vi "GUI_Pico8752_v2.vi"() -> ()   [LabVIEW 2020]
uses:
  Shared/GUI_Template/GUI_master/tcp_new_data_event.ctl
  Shared/GUI_Template/GUI_master/tcp new data cluster.ctl
panel:
  in  "StepSize\nDogleg":dbl=10.0
  in  "StepSize\nAMP1":dbl=100.0
  in  "StepSize\nPreAmp":dbl=30.0
  in  "StepSize\nXPW":dbl=5.0
  in  "Move Device 11 Neg":bool
  in  "Move Device 11 Pos":bool
  in  "Move Device 10 Pos":bool
  in  "Move Device 10 Neg":bool
  in  "Position.device 7::2":dbl caption="Position X" min=-10000.0 max=10000.0
  in  "Position.device 8::2":dbl caption="Position Y" min=-10000.0 max=10000.0
  in  "Move Device 8 Neg":bool
  in  "Move Device 8 Pos":bool
  in  "Move Device 7 Pos":bool
  in  "Move Device 7 Neg":bool
  in  "Position.device 4::2":dbl caption="Position X" min=-10000.0 max=10000.0
  in  "Position.device 5::2":dbl caption="Position Y" min=-10000.0 max=10000.0
  in  "Move Device 5 Neg":bool
  in  "Move Device 5 Pos":bool
  in  "Move Device 4 Pos":bool
  in  "Move Device 4 Neg":bool
  in  "Position.device 2::2":dbl caption="Position Y" min=-10000.0 max=10000.0
  in  "Move Device 1 Neg":bool
  in  "Move Device 1 Pos":bool
  in  "Move Device 2 Pos":bool
  in  "Move Device 2 Neg":bool
  in  "Position.device 10::2":dbl caption="Position X" min=-10000.0 max=10000.0
  in  "Position.device 11::2":dbl caption="Position Y" min=-10000.0 max=10000.0
  in  "Position.device 1::2":dbl caption="Position X" min=-10000.0 max=10000.0
  in  "GUIdevice 2":string="MCD-LT-PicoBooster"
  in  "stop":bool
  out "tcp data event":T1
  out "error IO 2":errorcluster
  # "XPW Input/\nBooster"
  # "PreAmp Input"
  # "Amp 1 Out"
  # "Dogleg"
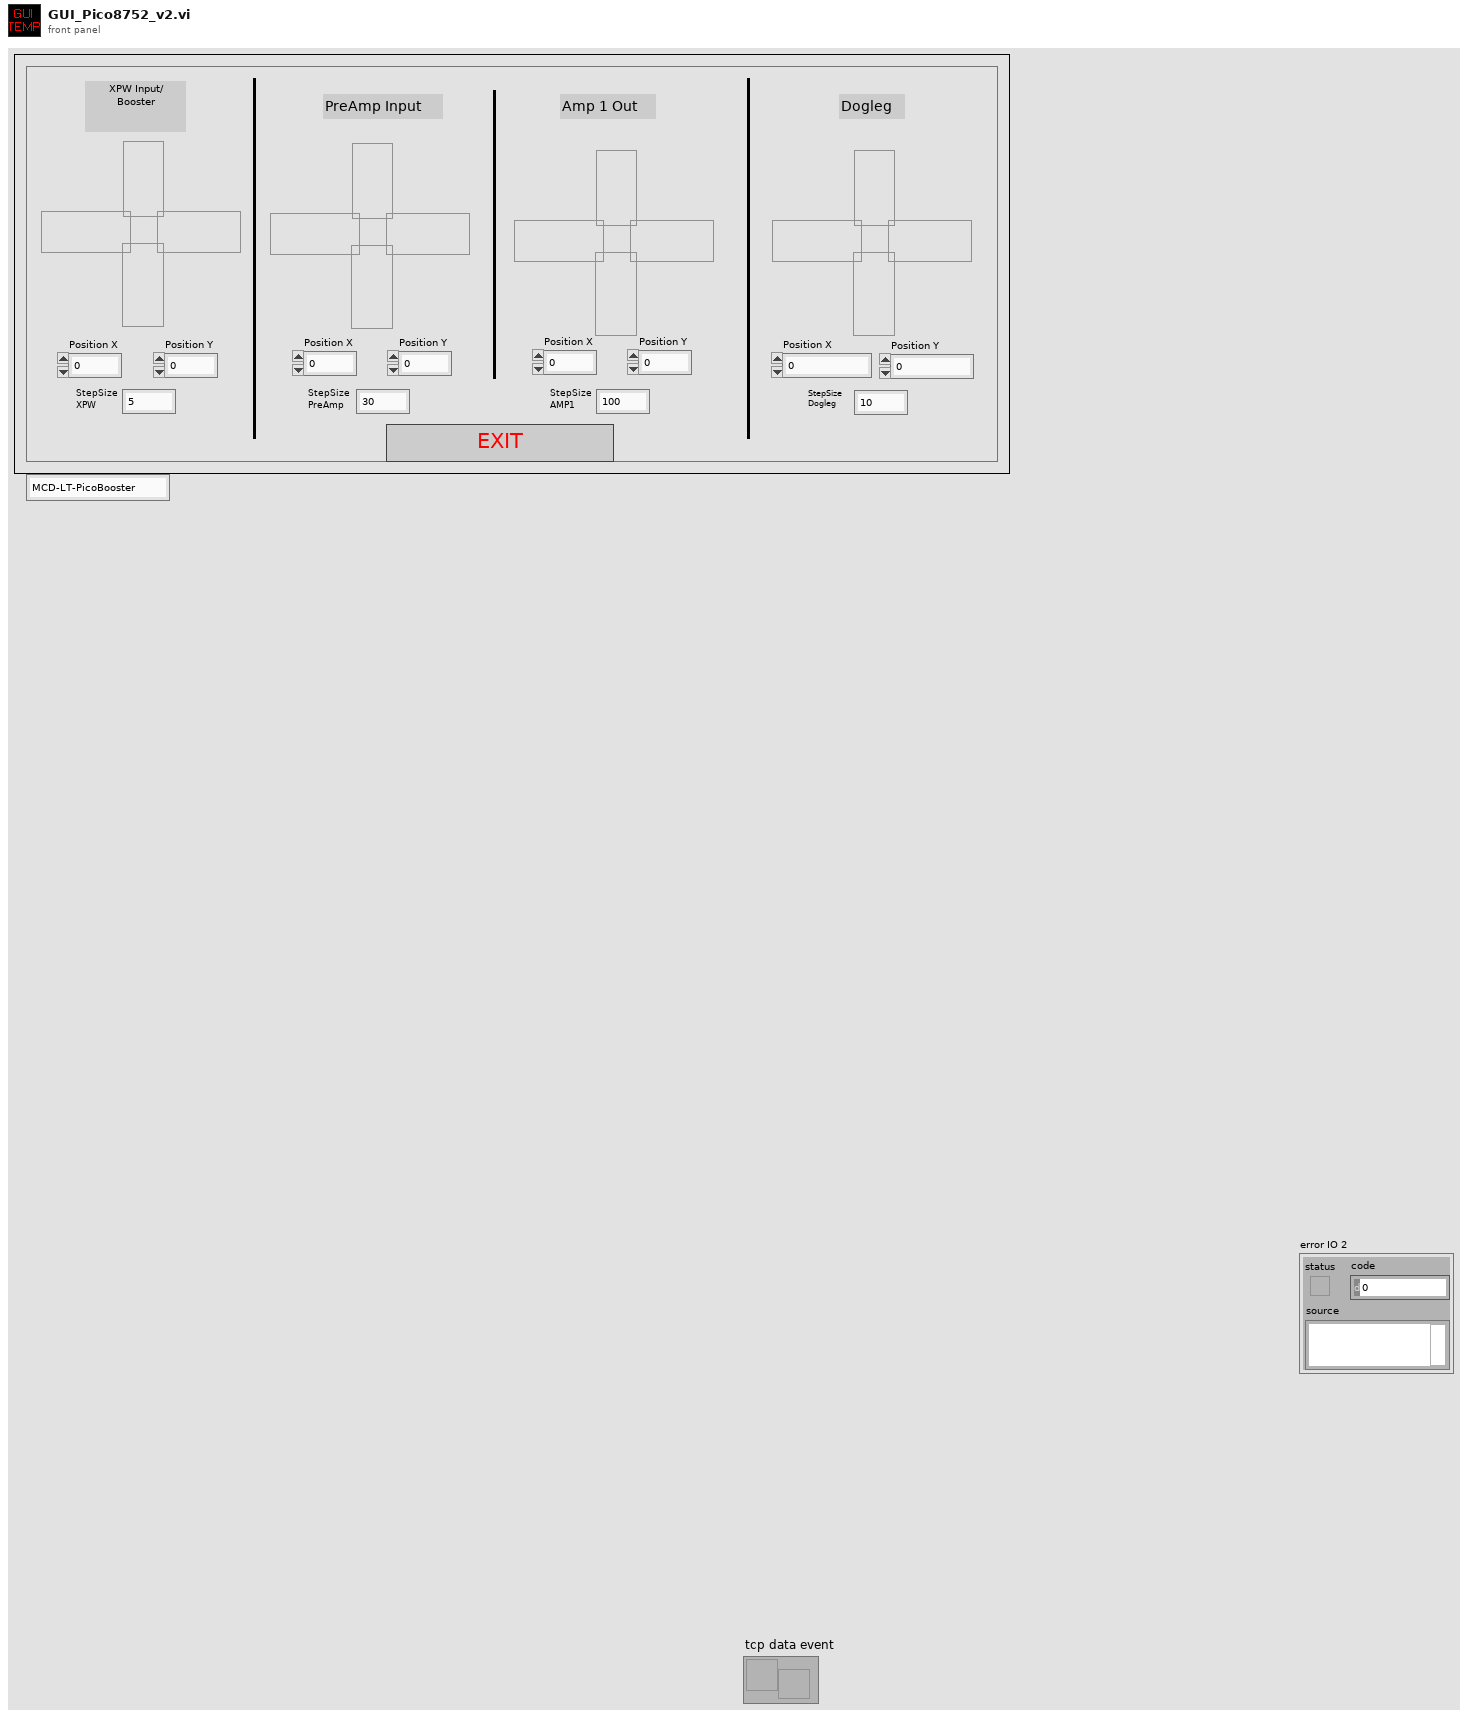
[diagram p1: front panel]
types:
  T1 = typedef "tcp_new_data_event.ctl" = refnum<user-event>
  T2 = typedef "tcp new data cluster.ctl" = cluster{"EventEnum":enum16{"new data", "connection status update"}, "Device name":string}
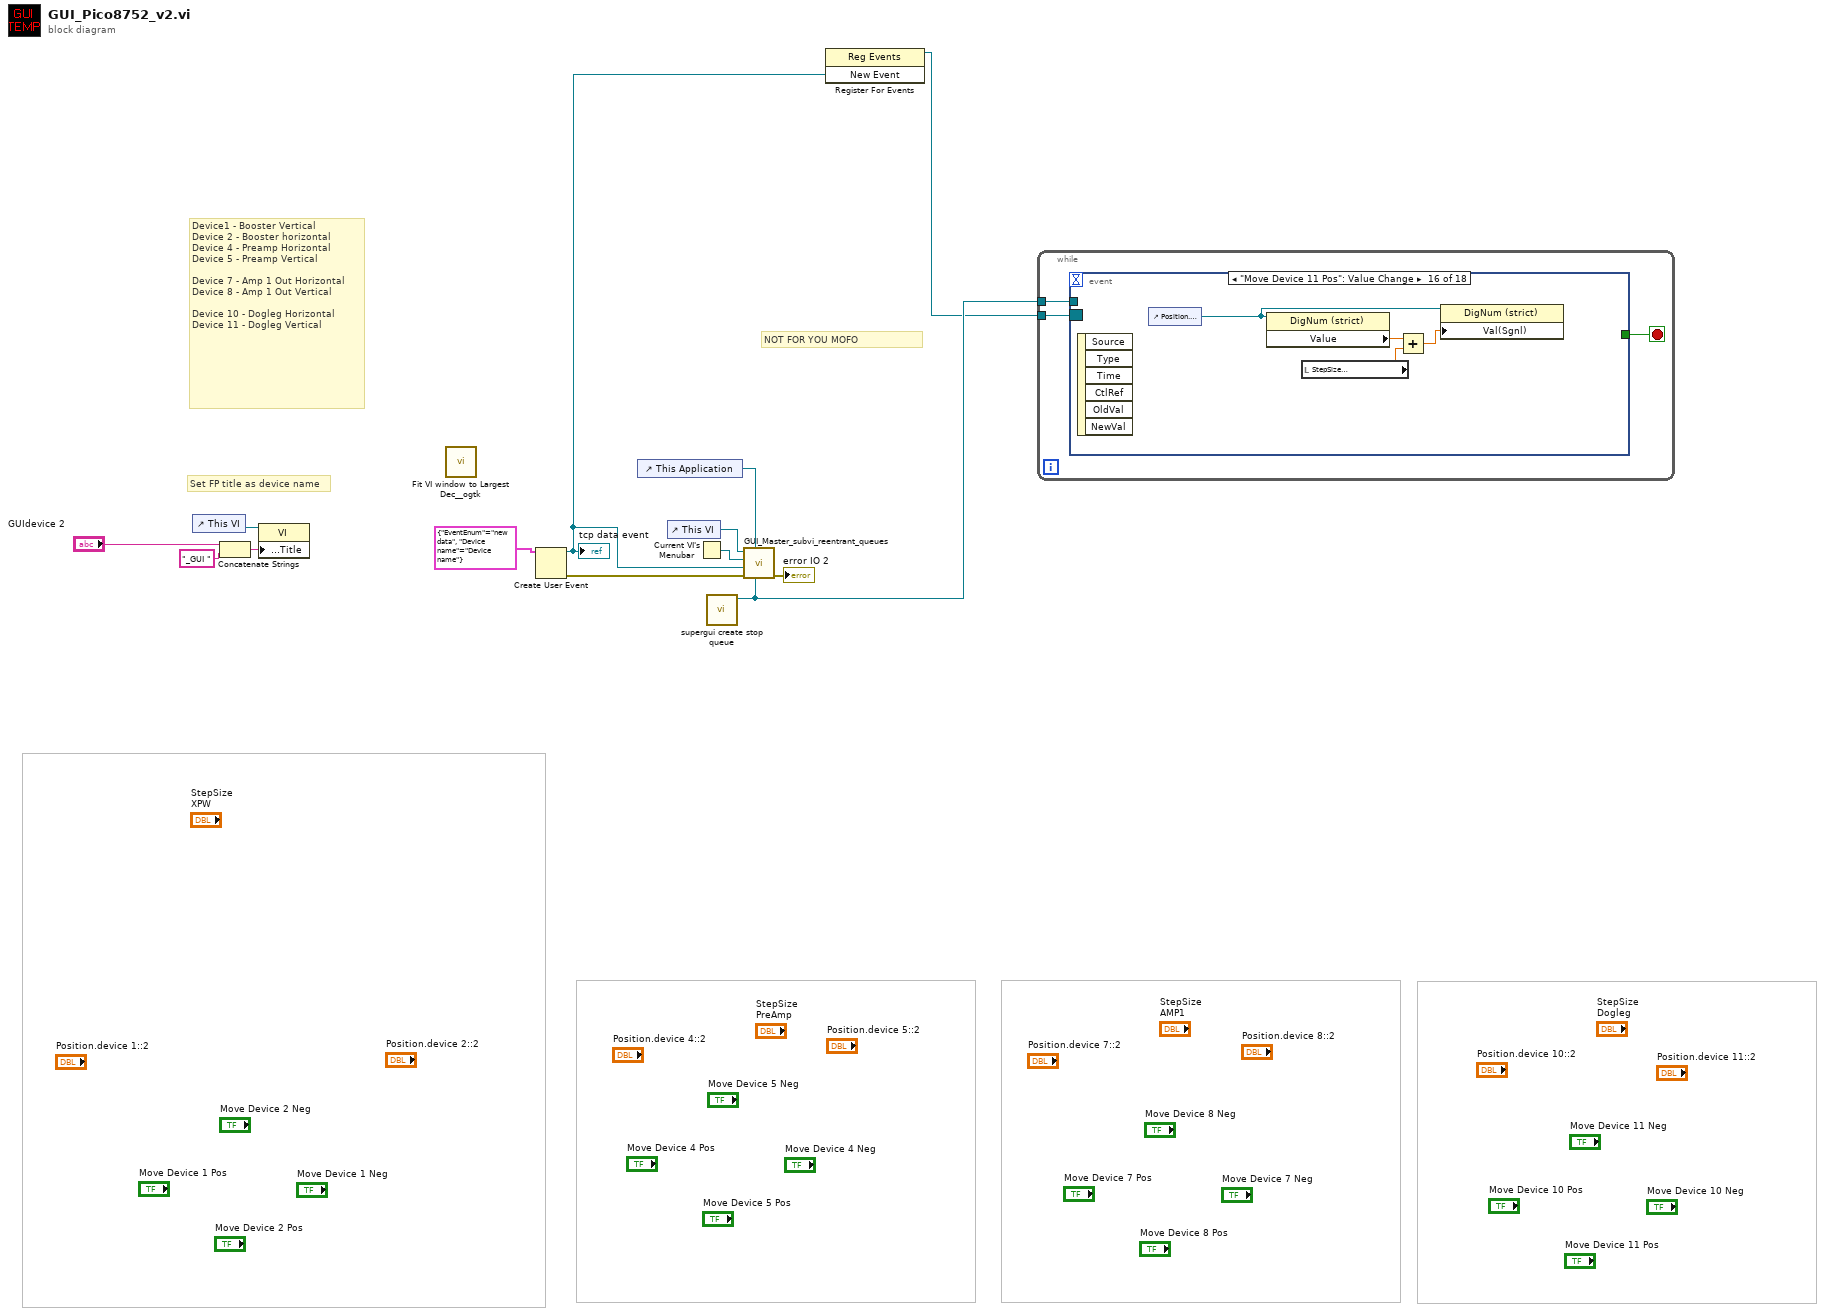
[diagram p0: block diagram]
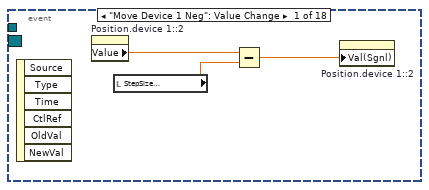
[diagram p2: hidden frame]
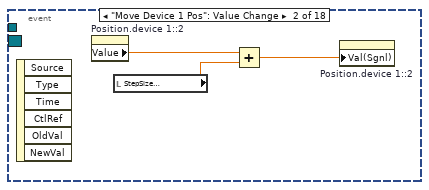
[diagram p3: hidden frame]
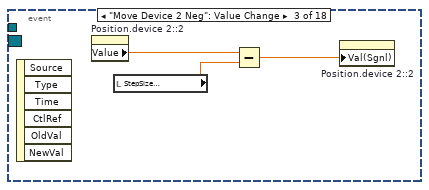
[diagram p4: hidden frame]
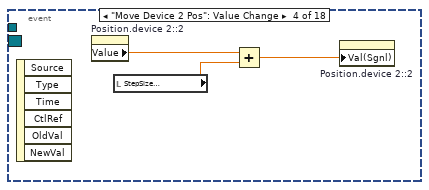
[diagram p5: hidden frame]
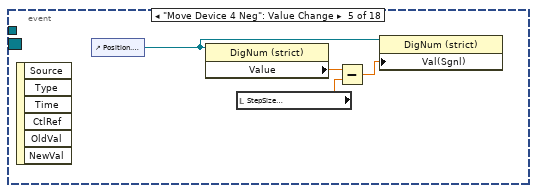
[diagram p6: hidden frame]
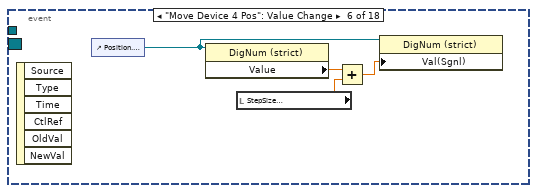
[diagram p7: hidden frame]
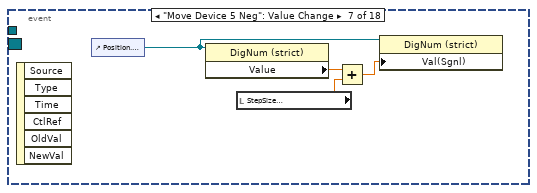
[diagram p8: hidden frame]
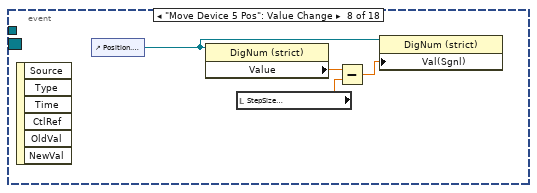
[diagram p9: hidden frame]
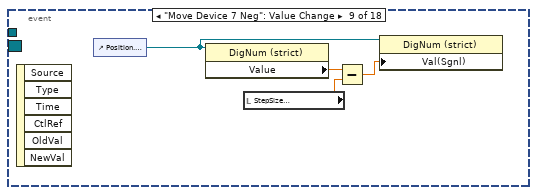
[diagram p10: hidden frame]
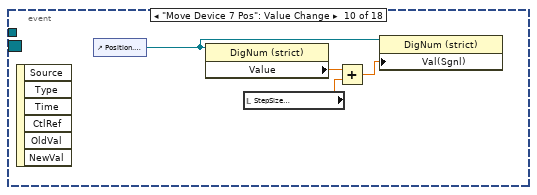
[diagram p11: hidden frame]
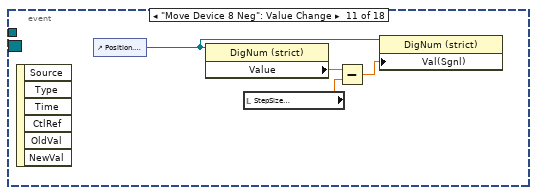
[diagram p12: hidden frame]
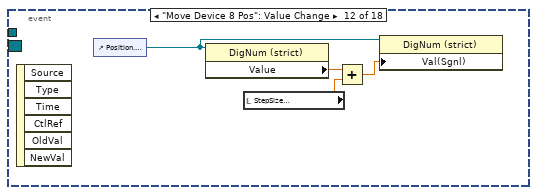
[diagram p13: hidden frame]
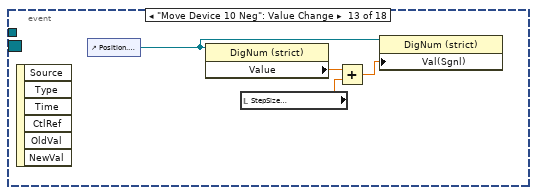
[diagram p14: hidden frame]
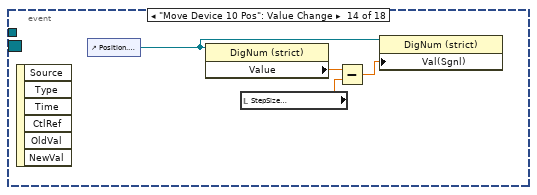
[diagram p15: hidden frame]
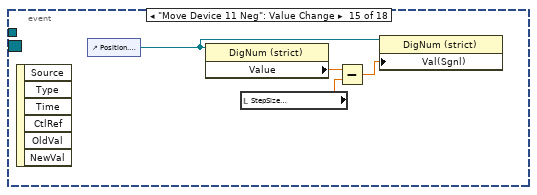
[diagram p16: hidden frame]
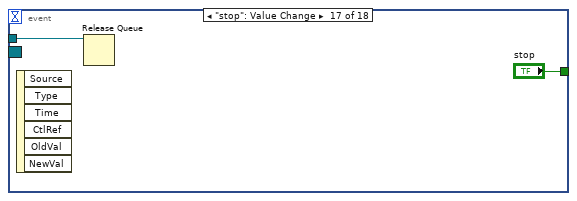
[diagram p17: hidden frame]
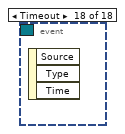
[diagram p18: hidden frame]
diagram:
  # "Device1 - Booster Vertical\nDevice 2 - Booster horizontal\nDevice 4 - Preamp Horizontal\nDevice 5 - Preamp Vertical\n\nDevice 7 - Amp 1 Out Horizontal\nDevice 8 - Amp 1 Out Vertical\n\nDevice 10 - Dogleg Horizontal\nDevice 11 - Dogleg Vertical"
  # "Set FP title as device name"
  # "NOT FOR YOU MOFO"
  n1 = control-ref of="This VI"() -> (w6:refnum<vi>)
  n2 = Concatenate Strings("GUIdevice 2", "_GUI ") -> (w5:string)
  n3 = property class="VI"(reference=w6, "Front Panel.Title"=w5) -> ()  [unwired: 1 in, 2 out]
  n4 = call <userlib>:"Fit VI window to Largest Dec__ogtk.vi"() -> ()  [unwired: 6 in, 2 out]
  n5 = Create User Event(user event datatype=T2 {"EventEnum"=enum."new data", "Device name"="Device name"} ("New Event")) -> (user event=w8:refnum<user-event>, error out=w9:errorcluster)  [unwired: 1 in]
  "tcp data event" <- w8
  n6 = control-ref of="This Application"() -> (w7:refnum<vi>)
  n7 = control-ref of="This VI"() -> (w12:refnum<vi>)
  n8 = Current VI's Menubar() -> (w11:refnum<k9>)
  n9 = call "supergui create stop queue.vi"() -> ("STOP Queue out"=w2:refnum<queue>)  [unwired: 11 in]
  n10 = call "GUI_Master_subvi_reentrant_queues.vi"("STOP Queue in"=w2, "This Application"=w7, "error in (no error)"=w9, "tcp data event"=w8, "Caller menu reference"=w11, "Caller VI ref"=w12) -> ("error out"=→"error IO 2":errorcluster)  [unwired: 5 in]
  n11 = register-events(w8) -> (reference out=w1:refnum<event-registration>)  [unwired: 2 in, 1 out]
  n12 = while {
    tunnel: w2 -> [w15]
    tunnel: w1 -> [w14]
    stop <- w16 stop-if-true
    n13 = event shown="[15] \"Move Device 11 Pos\": Value Change" {
      selector: w14 -> [_ _ _ _ _ _ _ _ _ _ _ _ _ _ _ _ _ _]
      dyn-events: _ -> [_ _ _ _ _ _ _ _ _ _ _ _ _ _ _ _ _ _]
      timeout: _ -> [_ _ _ _ _ _ _ _ _ _ _ _ _ _ _ _ _ _]
      tunnel: [_ _ _ _ _ _ _ _ _ _ _ _ _ _ _ _ "stop" _] -> w16
      tunnel: w15 -> [_ _ _ _ _ _ _ _ _ _ _ _ _ _ _ _ w77 _]
      event "Move Device 1 Neg": Value Change {
        n14 = event-data() -> ()  [unwired: 1 in, 6 out]
        n15 = property on="Position.device 1::2" class="DigNum (strict)"() -> ("Value"=w18:dbl)  [unwired: 2 in, 2 out]
        n16 = local read "StepSize\nXPW"() -> (w19:dbl)
        n17 = Subtract(x=w18, y=w19) -> (x-y=w17:dbl)
        n18 = property on="Position.device 1::2" class="DigNum (strict)"("Val(Sgnl)"=w17) -> ()  [unwired: 2 in, 2 out]
      }
      event "Move Device 1 Pos": Value Change {
        n19 = event-data() -> ()  [unwired: 1 in, 6 out]
        n20 = property on="Position.device 1::2" class="DigNum (strict)"() -> ("Value"=w21:dbl)  [unwired: 2 in, 2 out]
        n21 = local read "StepSize\nXPW"() -> (w22:dbl)
        n22 = Add(x=w21, y=w22) -> (x+y=w20:dbl)
        n23 = property on="Position.device 1::2" class="DigNum (strict)"("Val(Sgnl)"=w20) -> ()  [unwired: 2 in, 2 out]
      }
      event "Move Device 2 Neg": Value Change {
        n24 = event-data() -> ()  [unwired: 1 in, 6 out]
        n25 = property on="Position.device 2::2" class="DigNum (strict)"() -> ("Value"=w24:dbl)  [unwired: 2 in, 2 out]
        n26 = local read "StepSize\nXPW"() -> (w25:dbl)
        n27 = Subtract(x=w24, y=w25) -> (x-y=w23:dbl)
        n28 = property on="Position.device 2::2" class="DigNum (strict)"("Val(Sgnl)"=w23) -> ()  [unwired: 2 in, 2 out]
      }
      event "Move Device 2 Pos": Value Change {
        n29 = event-data() -> ()  [unwired: 1 in, 6 out]
        n30 = property on="Position.device 2::2" class="DigNum (strict)"() -> ("Value"=w27:dbl)  [unwired: 2 in, 2 out]
        n31 = local read "StepSize\nXPW"() -> (w28:dbl)
        n32 = Add(x=w27, y=w28) -> (x+y=w26:dbl)
        n33 = property on="Position.device 2::2" class="DigNum (strict)"("Val(Sgnl)"=w26) -> ()  [unwired: 2 in, 2 out]
      }
      event "Move Device 4 Neg": Value Change {
        n34 = event-data() -> ()  [unwired: 1 in, 6 out]
        n35 = control-ref of="Position.device 4::2"() -> (w29:refnum<vi>)
        n36 = property on="Property Node" class="DigNum (strict)"(reference=w29) -> ("Value"=w31:dbl)  [unwired: 1 in, 2 out]
        n37 = local read "StepSize\nPreAmp"() -> (w32:dbl)
        n38 = Subtract(x=w31, y=w32) -> (x-y=w30:dbl)
        n39 = property on="Property Node" class="DigNum (strict)"(reference=w29, "Val(Sgnl)"=w30) -> ()  [unwired: 1 in, 2 out]
      }
      event "Move Device 4 Pos": Value Change {
        n40 = event-data() -> ()  [unwired: 1 in, 6 out]
        n41 = control-ref of="Position.device 4::2"() -> (w33:refnum<vi>)
        n42 = property on="Property Node" class="DigNum (strict)"(reference=w33) -> ("Value"=w35:dbl)  [unwired: 1 in, 2 out]
        n43 = local read "StepSize\nPreAmp"() -> (w36:dbl)
        n44 = Add(x=w35, y=w36) -> (x+y=w34:dbl)
        n45 = property on="Property Node" class="DigNum (strict)"(reference=w33, "Val(Sgnl)"=w34) -> ()  [unwired: 1 in, 2 out]
      }
      event "Move Device 5 Neg": Value Change {
        n46 = event-data() -> ()  [unwired: 1 in, 6 out]
        n47 = control-ref of="Position.device 5::2"() -> (w37:refnum<vi>)
        n48 = property on="Property Node" class="DigNum (strict)"(reference=w37) -> ("Value"=w39:dbl)  [unwired: 1 in, 2 out]
        n49 = local read "StepSize\nPreAmp"() -> (w40:dbl)
        n50 = Add(x=w39, y=w40) -> (x+y=w38:dbl)
        n51 = property on="Property Node" class="DigNum (strict)"(reference=w37, "Val(Sgnl)"=w38) -> ()  [unwired: 1 in, 2 out]
      }
      event "Move Device 5 Pos": Value Change {
        n52 = event-data() -> ()  [unwired: 1 in, 6 out]
        n53 = control-ref of="Position.device 5::2"() -> (w41:refnum<vi>)
        n54 = property on="Property Node" class="DigNum (strict)"(reference=w41) -> ("Value"=w43:dbl)  [unwired: 1 in, 2 out]
        n55 = local read "StepSize\nPreAmp"() -> (w44:dbl)
        n56 = Subtract(x=w43, y=w44) -> (x-y=w42:dbl)
        n57 = property on="Property Node" class="DigNum (strict)"(reference=w41, "Val(Sgnl)"=w42) -> ()  [unwired: 1 in, 2 out]
      }
      event "Move Device 7 Neg": Value Change {
        n58 = event-data() -> ()  [unwired: 1 in, 6 out]
        n59 = control-ref of="Position.device 7::2"() -> (w45:refnum<vi>)
        n60 = property on="Property Node" class="DigNum (strict)"(reference=w45) -> ("Value"=w47:dbl)  [unwired: 1 in, 2 out]
        n61 = local read "StepSize\nAMP1"() -> (w48:dbl)
        n62 = Subtract(x=w47, y=w48) -> (x-y=w46:dbl)
        n63 = property on="Property Node" class="DigNum (strict)"(reference=w45, "Val(Sgnl)"=w46) -> ()  [unwired: 1 in, 2 out]
      }
      event "Move Device 7 Pos": Value Change {
        n64 = event-data() -> ()  [unwired: 1 in, 6 out]
        n65 = control-ref of="Position.device 7::2"() -> (w49:refnum<vi>)
        n66 = property on="Property Node" class="DigNum (strict)"(reference=w49) -> ("Value"=w51:dbl)  [unwired: 1 in, 2 out]
        n67 = local read "StepSize\nAMP1"() -> (w52:dbl)
        n68 = Add(x=w51, y=w52) -> (x+y=w50:dbl)
        n69 = property on="Property Node" class="DigNum (strict)"(reference=w49, "Val(Sgnl)"=w50) -> ()  [unwired: 1 in, 2 out]
      }
      event "Move Device 8 Neg": Value Change {
        n70 = event-data() -> ()  [unwired: 1 in, 6 out]
        n71 = control-ref of="Position.device 8::2"() -> (w53:refnum<vi>)
        n72 = property on="Property Node" class="DigNum (strict)"(reference=w53) -> ("Value"=w55:dbl)  [unwired: 1 in, 2 out]
        n73 = local read "StepSize\nAMP1"() -> (w56:dbl)
        n74 = Subtract(x=w55, y=w56) -> (x-y=w54:dbl)
        n75 = property on="Property Node" class="DigNum (strict)"(reference=w53, "Val(Sgnl)"=w54) -> ()  [unwired: 1 in, 2 out]
      }
      event "Move Device 8 Pos": Value Change {
        n76 = event-data() -> ()  [unwired: 1 in, 6 out]
        n77 = control-ref of="Position.device 8::2"() -> (w57:refnum<vi>)
        n78 = property on="Property Node" class="DigNum (strict)"(reference=w57) -> ("Value"=w59:dbl)  [unwired: 1 in, 2 out]
        n79 = local read "StepSize\nAMP1"() -> (w60:dbl)
        n80 = Add(x=w59, y=w60) -> (x+y=w58:dbl)
        n81 = property on="Property Node" class="DigNum (strict)"(reference=w57, "Val(Sgnl)"=w58) -> ()  [unwired: 1 in, 2 out]
      }
      event "Move Device 10 Neg": Value Change {
        n82 = event-data() -> ()  [unwired: 1 in, 6 out]
        n83 = control-ref of="Position.device 10::2"() -> (w61:refnum<vi>)
        n84 = property on="Property Node" class="DigNum (strict)"(reference=w61) -> ("Value"=w63:dbl)  [unwired: 1 in, 2 out]
        n85 = local read "StepSize\nDogleg"() -> (w64:dbl)
        n86 = Add(x=w63, y=w64) -> (x+y=w62:dbl)
        n87 = property on="Property Node" class="DigNum (strict)"(reference=w61, "Val(Sgnl)"=w62) -> ()  [unwired: 1 in, 2 out]
      }
      event "Move Device 10 Pos": Value Change {
        n88 = event-data() -> ()  [unwired: 1 in, 6 out]
        n89 = control-ref of="Position.device 10::2"() -> (w65:refnum<vi>)
        n90 = property on="Property Node" class="DigNum (strict)"(reference=w65) -> ("Value"=w67:dbl)  [unwired: 1 in, 2 out]
        n91 = local read "StepSize\nDogleg"() -> (w68:dbl)
        n92 = Subtract(x=w67, y=w68) -> (x-y=w66:dbl)
        n93 = property on="Property Node" class="DigNum (strict)"(reference=w65, "Val(Sgnl)"=w66) -> ()  [unwired: 1 in, 2 out]
      }
      event "Move Device 11 Neg": Value Change {
        n94 = event-data() -> ()  [unwired: 1 in, 6 out]
        n95 = control-ref of="Position.device 11::2"() -> (w69:refnum<vi>)
        n96 = property on="Property Node" class="DigNum (strict)"(reference=w69) -> ("Value"=w71:dbl)  [unwired: 1 in, 2 out]
        n97 = local read "StepSize\nDogleg"() -> (w72:dbl)
        n98 = Subtract(x=w71, y=w72) -> (x-y=w70:dbl)
        n99 = property on="Property Node" class="DigNum (strict)"(reference=w69, "Val(Sgnl)"=w70) -> ()  [unwired: 1 in, 2 out]
      }
      event "Move Device 11 Pos": Value Change {
        n100 = event-data() -> ()  [unwired: 1 in, 6 out]
        n101 = control-ref of="Position.device 11::2"() -> (w73:refnum<vi>)
        n102 = property on="Property Node" class="DigNum (strict)"(reference=w73) -> ("Value"=w75:dbl)  [unwired: 1 in, 2 out]
        n103 = local read "StepSize\nDogleg"() -> (w76:dbl)
        n104 = Add(x=w75, y=w76) -> (x+y=w74:dbl)
        n105 = property on="Property Node" class="DigNum (strict)"(reference=w73, "Val(Sgnl)"=w74) -> ()  [unwired: 1 in, 2 out]
      }
      event "stop": Value Change {
        n106 = event-data() -> ()  [unwired: 1 in, 6 out]
        n107 = Release Queue(queue=w77) -> ()  [unwired: 2 in, 3 out]
      }
      event Timeout {
        n108 = event-data() -> ()  [unwired: 1 in, 3 out]
      }
    }
  }
